vi "OnButtonSingle.vi"(0 "Input":bool) -> (1 "Pressed":bool, 2 "Released":bool)   [LabVIEW 2016]
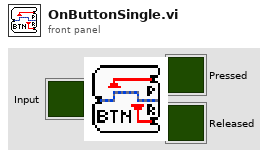
[diagram p1: front panel]
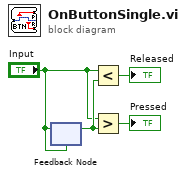
[diagram p0: block diagram]
diagram:
  n1 = feedback-in #1("Input") -> ()
  n2 = feedback #1("Input") -> (w3:bool)
  n3 = Less?(x="Input", y=w3) -> (x < y?=→"Released":bool)
  n4 = Greater?(x="Input", y=w3) -> (0:→"Pressed":bool)
